vi "USB2XXXOpenbusTest.vi"() -> ()   [LabVIEW 2010]
uses:
  PublicFiles/USB2XXX.dll
panel:
  in  "pReadData":T1
  out "pReadData out":T1
  in  "pWriteData":T2
  in  "Channel Index":i32(ring) items=["CH0", "CH1", "CH2", "CH3", "CH4", "CH5", "CH6", "CH7"]
  in  "Device Index":i32(ring) items=["0", "1", "2", "3", "4", "5"]
  out "Flag(T:Write;F:Read)":bool=TRUE
  in  "stop":bool
  in  "Read":bool
  in  "Write":bool
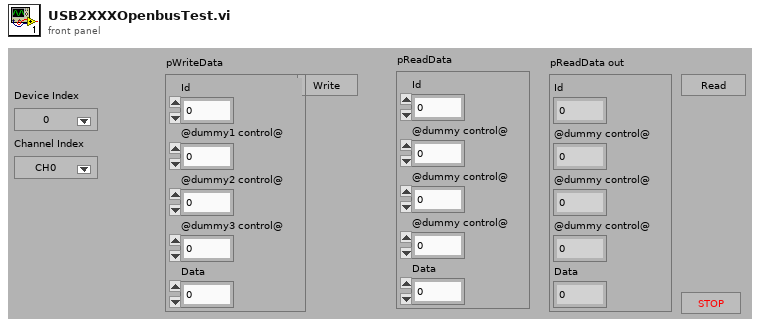
[diagram p1: front panel]
types:
  T1 = cluster{"Id":i8, "@dummy control@":i8, "@dummy control@":i8, "@dummy control@":i8, "Data":u32}
  T2 = cluster{"Id":i8, "@dummy1 control@":i8, "@dummy2 control@":i8, "@dummy3 control@":i8, "Data":u32}
  T3 = cluster{"Id":i8, "@dummy control@":i8, "@dummy control@":i8, "@dummy control@":i8, "Data":u32}[]
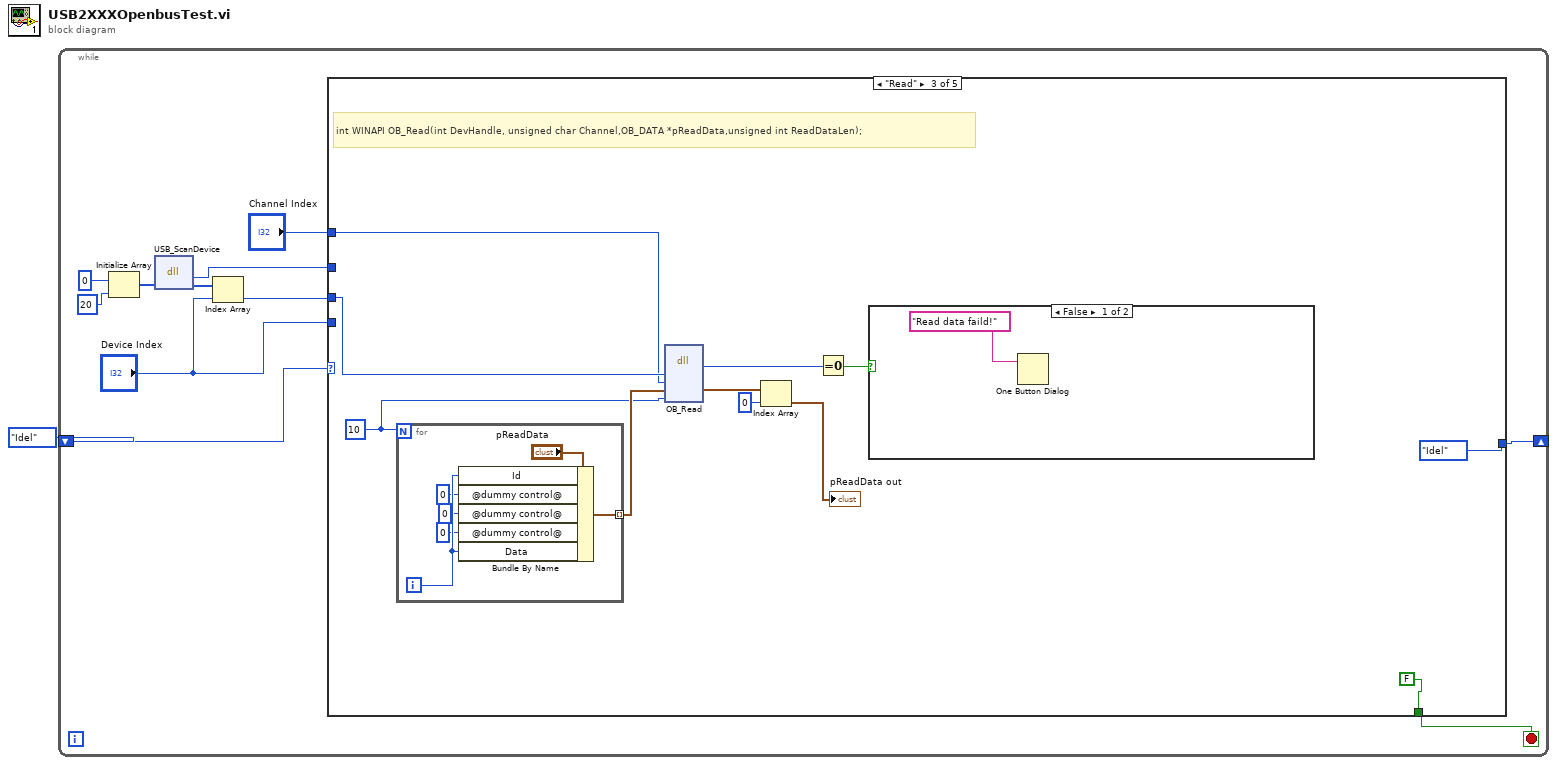
[diagram p0: block diagram]
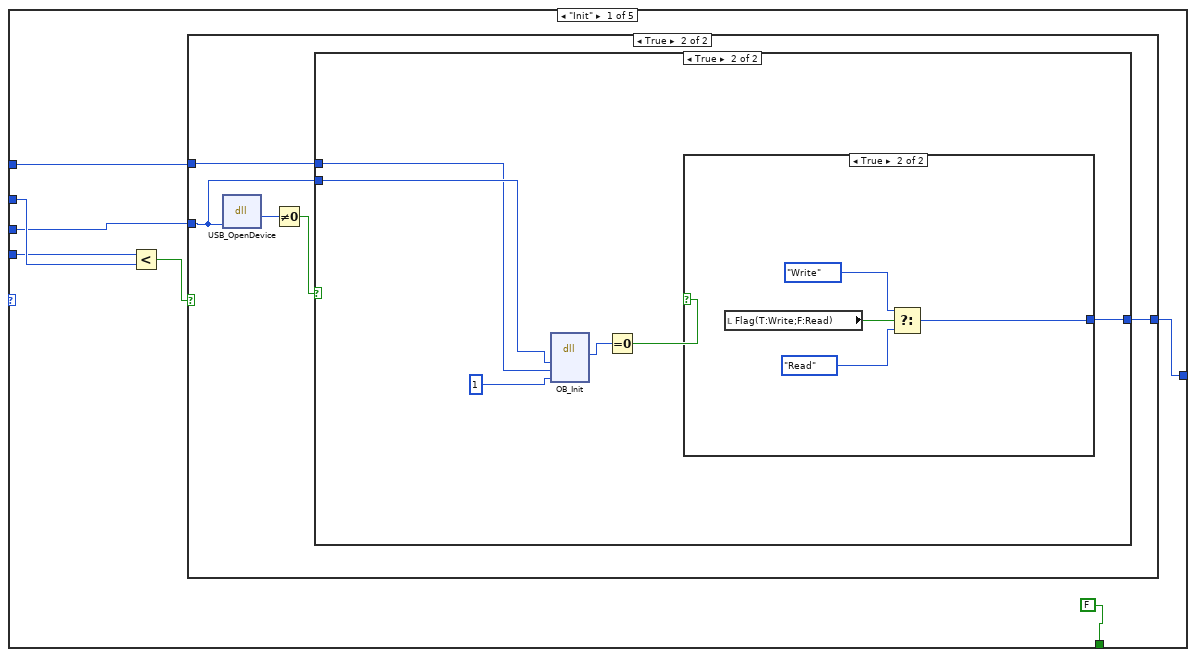
[diagram p2: hidden frame]
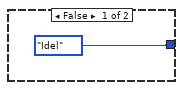
[diagram p3: hidden frame]
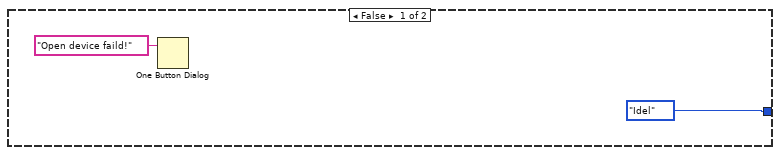
[diagram p4: hidden frame]
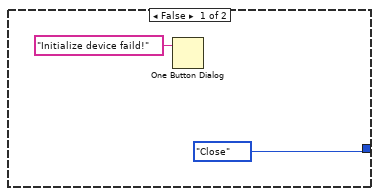
[diagram p5: hidden frame]
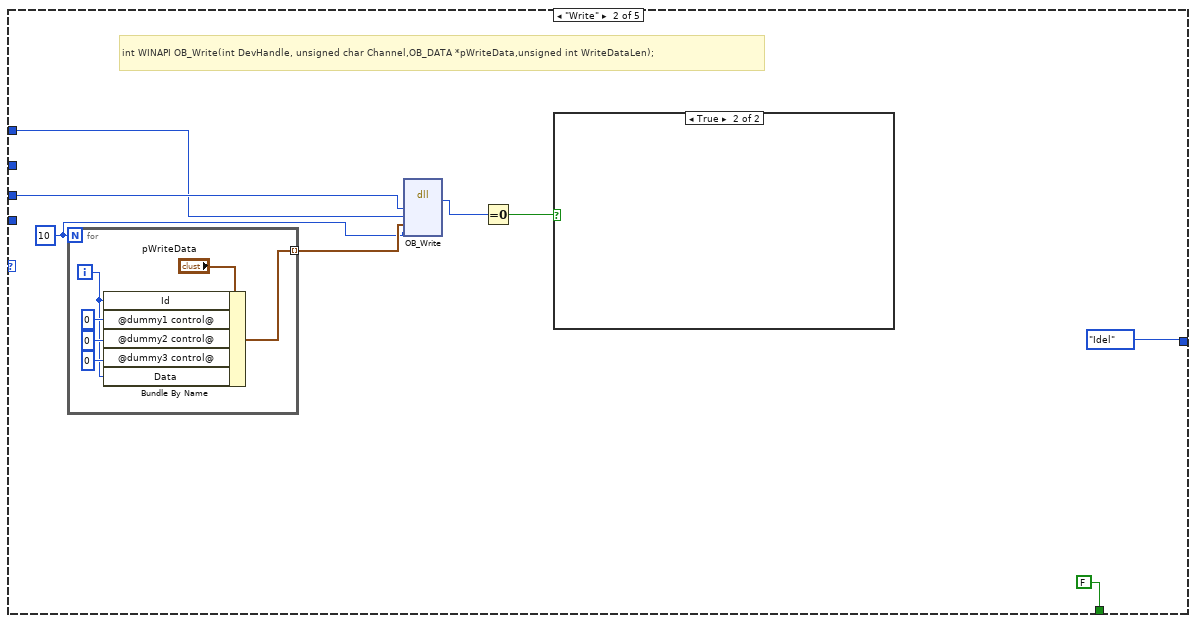
[diagram p6: hidden frame]
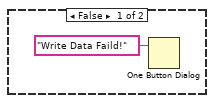
[diagram p7: hidden frame]
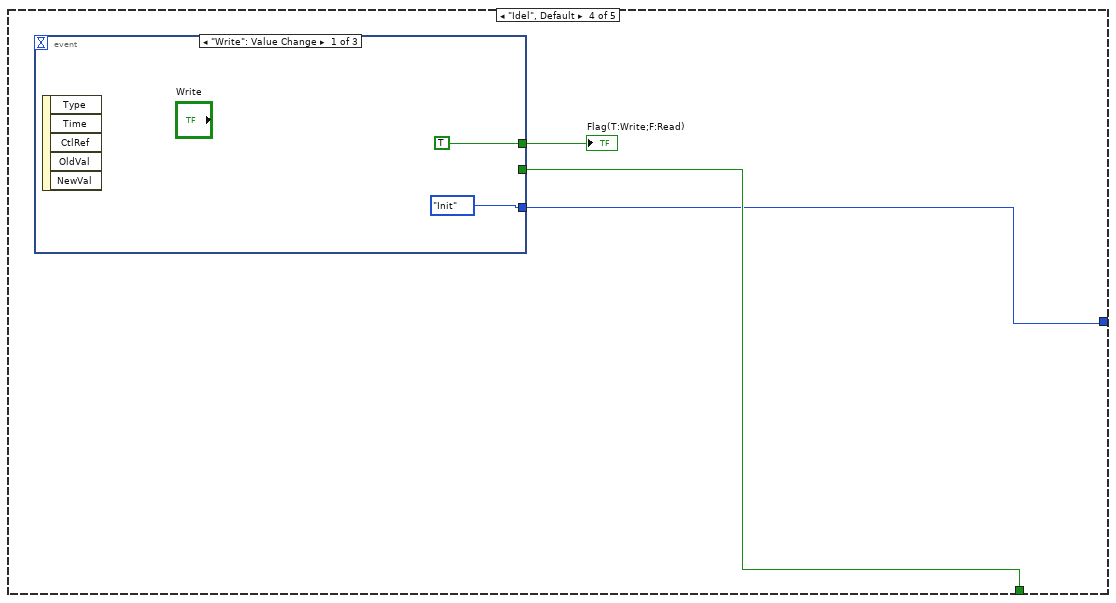
[diagram p9: hidden frame]
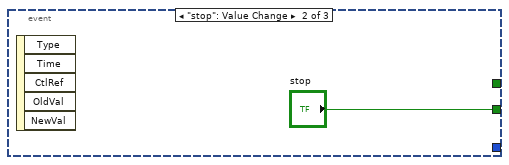
[diagram p10: hidden frame]
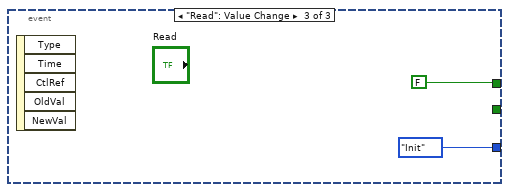
[diagram p11: hidden frame]
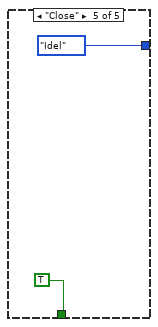
[diagram p12: hidden frame]
diagram:
  n1 = while {
    shift-right: [w11] -> _
    shift-left: enum16{"Init", "Write", "Read", "Idel", "Close"}."Idel" ("Enum") -> [w12]
    stop <- w9 stop-if-true
    n2 = Initialize Array(0, 20 ("dimension size")) -> (w8:i32[])
    n3 = dll-call lib="F:/OtherWork/STM32/USB2XXX_Example/trunk/Labview/PublicFiles/USB2XXX.dll" fn="USB_ScanDevice"("pDevNum"=w8) -> ("return type"=w3:i32, "pDevNum"=w5:i32[])  [unwired: 3 in, 2 out]
    n4 = Index Array(array=w5, index="Device Index") -> (element=w4:i32)
    n5 = case shown="\"Read\"" w12 {
      tunnel: [w18 enum16{"Init", "Write", "Read", "Idel", "Close"}."Idel" ("Enum") enum16{"Init", "Write", "Read", "Idel", "Close"}."Idel" ("Enum") w73 enum16{"Init", "Write", "Read", "Idel", "Close"}."Idel" ("Enum")] -> w11
      tunnel: w4 -> [w14 w44 w62 _ _]
      tunnel: "Channel Index" -> [w17 w43 w61 _ _]
      tunnel: [FALSE FALSE FALSE w74 TRUE] -> w9
      tunnel: w3 -> [w15 _ _ _ _]
      tunnel: "Device Index" -> [w13 _ _ _ _]
      frame "Init" {
        n6 = Less?(x=w13, y=w15) -> (x < y?=w19:bool)
        n7 = case shown="True" w19 {
          tunnel: w14 -> [_ w22]
          tunnel: w17 -> [_ w23]
          tunnel: [enum16{"Init", "Write", "Read", "Idel", "Close"}."Idel" ("Enum") w21] -> w18
          frame False {
          }
          frame True {
            n8 = dll-call lib="F:/OtherWork/STM32/USB2XXX_Example/trunk/Labview/PublicFiles/USB2XXX.dll" fn="USB_OpenDevice"("DevIndex"=w22) -> ("return type"=w25:u8)  [unwired: 4 in, 2 out]
            n9 = Not Equal To 0?(x=w25) -> (x != 0?=w24:bool)
            n10 = case shown="True" w24 {
              tunnel: w23 -> [_ w30]
              tunnel: w22 -> [_ w31]
              tunnel: [enum16{"Init", "Write", "Read", "Idel", "Close"}."Idel" ("Enum") w32] -> w21
              frame False {
                n11 = One Button Dialog(message="Open device faild!") -> ()  [unwired: 1 in, 1 out]
              }
              frame True {
                n12 = dll-call lib="F:/OtherWork/STM32/USB2XXX_Example/trunk/Labview/PublicFiles/USB2XXX.*" fn="OB_Init"("DevHandle"=w31, "Channel"=w30, "EnInternalPull"=u8 1 ("OwnAddr")) -> (w28:i32)  [unwired: 6 in, 2 out]
                n13 = Equal To 0?(x=w28) -> (x = 0?=w33:bool)
                n14 = case shown="True" w33 {
                  tunnel: [enum16{"Init", "Write", "Read", "Idel", "Close"}."Close" ("Enum") w36] -> w32
                  frame False {
                    n15 = One Button Dialog(message="Initialize device faild!") -> ()  [unwired: 1 in, 1 out]
                  }
                  frame True {
                    n16 = local read "Flag(T:Write;F:Read)"() -> (w39:bool)
                    n17 = Select(t=enum16{"Init", "Write", "Read", "Idel", "Close"}."Write" ("Enum"), s=w39, f=enum16{"Init", "Write", "Read", "Idel", "Close"}."Read" ("Enum")) -> (s? t:f=w36:enum16{"Init", "Write", "Read", "Idel", "Close"})
                  }
                }
              }
            }
          }
        }
      }
      frame "Write" {
        w40 = 10 ("dimension size")
        # "int WINAPI OB_Write(int DevHandle, unsigned char Channel,OB_DATA *pWriteData,unsigned int WriteDataLen);"
        n18 = for {
          N: w40 -> [_]
          tunnel: [w52] -> w41 mode=indexing
          i -> [w48]
          n19 = Bundle By Name(cluster="pWriteData", "Id"=w48, "@dummy1 control@"=i8 0, "@dummy2 control@"=i8 0, "@dummy3 control@"=i8 0, "Data"=w48) -> (w52:T2)
        }
        n20 = dll-call lib="F:/OtherWork/STM32/USB2XXX_Example/trunk/Labview/PublicFiles/USB2XXX.dll" fn="OB_Write"("DevHandle"=w44, "Channel"=w43, "pWriteData"=w41, "WriteDataLen"=w40) -> ("return type"=w42:i32)  [unwired: 7 in, 2 out]
        n21 = Equal To 0?(x=w42) -> (x = 0?=w47:bool)
        n22 = case shown="True" w47 {
          frame False {
            n23 = One Button Dialog(message="Write Data Faild!") -> ()  [unwired: 1 in, 1 out]
          }
          frame True {
          }
        }
      }
      frame "Read" {
        w58 = u32 10 ("ReadDataLen")
        # "int WINAPI OB_Read(int DevHandle, unsigned char Channel,OB_DATA *pReadData,unsigned int ReadDataLen);"
        n24 = for {
          N: w58 -> [_]
          tunnel: [w69] -> w59 mode=indexing
          i -> [w70]
          n25 = Bundle By Name(cluster="pReadData", "Id"=w70, "@dummy control@"=i8 0, "@dummy control@"=i8 0, "@dummy control@"=i8 0, "Data"=w70) -> (w69:T1)
        }
        n26 = dll-call lib="F:/OtherWork/STM32/USB2XXX_Example/trunk/Labview/PublicFiles/USB2XXX.dll" fn="OB_Read"("DevHandle"=w62, "Channel"=w61, "pReadData"=w59, "ReadDataLen"=w58) -> ("return type"=w60:i32, "pReadData"=w57:T3)  [unwired: 6 in, 2 out]
        n27 = Index Array(array=w57, index=0) -> (element=→"pReadData out":T1)
        n28 = Equal To 0?(x=w60) -> (x = 0?=w65:bool)
        n29 = case shown="False" w65 {
          frame False {
            n30 = One Button Dialog(message="Read data faild!") -> ()  [unwired: 1 in, 1 out]
          }
          frame True {
          }
        }
      }
      frame "Idel", Default {
        n31 = event shown="[0] \"Write\": Value Change" {
          selector: _ -> [_ _ _]
          dyn-events: _ -> [_ _ _]
          timeout: _ -> [_ _ _]
          tunnel: [TRUE _ FALSE] -> w75
          tunnel: [_ "stop" _] -> w74
          tunnel: [enum16{"Init", "Write", "Read", "Idel", "Close"}."Init" ("Enum") _ enum16{"Init", "Write", "Read", "Idel", "Close"}."Init" ("Enum")] -> w73
          event "Write": Value Change {
            n32 = event-data() -> ()  [unwired: 1 in, 5 out]
          }
          event "stop": Value Change {
            n33 = event-data() -> ()  [unwired: 1 in, 5 out]
          }
          event "Read": Value Change {
            n34 = event-data() -> ()  [unwired: 1 in, 5 out]
          }
        }
        "Flag(T:Write;F:Read)" <- w75
      }
      frame "Close" {
      }
    }
  }
